vi "Autonomous Independent.vi"   [LabVIEW 2019]
doc: "This VI is called when autonomous begins, and will automatically be terminated when autonomous ends. You can carry out timed or sensor driven robot movement independently without needing to return to the caller."
uses:
  <vilib>/Utility/file.llb/Read Delimited Spreadsheet (string).vi
  RobotGlobal.vi
  Classes/Robot/Panzer/Panzer.lvclass
panel:
  # "Be sure to right-click and choose Data Operations>>Make Current Value default if you want to save the array values with the VI"
types:
  T1 = typedef "RobotObjects.ctl" = cluster{"Drive.lvclass":refnum<class "Tank Drive.lvclass">, "Pneumatics.lvclass":refnum<class "Pneumatics.lvclass">, "Vision.lvclass":refnum<class "Vision.lvclass">, "Joysticks.lvclass":refnum<class "Joysticks.lvclass">, "Elevator.lvclass":refnum<class "Elevator.lvclass">, "Hatch.lvclass":refnum<class "Hatch.lvclass">, "Cargo.lvclass":refnum<class "Cargo.lvclass">, "DriveOld.lvclass":refnum<class "Drive.lvclass">, "Robot.lvclass":refnum<class "Robot.lvclass">, "Control Panel.lvclass":refnum<class "Control Panel.lvclass">, "Climber.lvclass":refnum<class "Climber.lvclass">, "Turret.lvlib:Turret.lvclass":refnum<class "Turret.lvclass">, "Power Cell Handler.lvclass":refnum<class "Power Cell Handler.lvclass">}
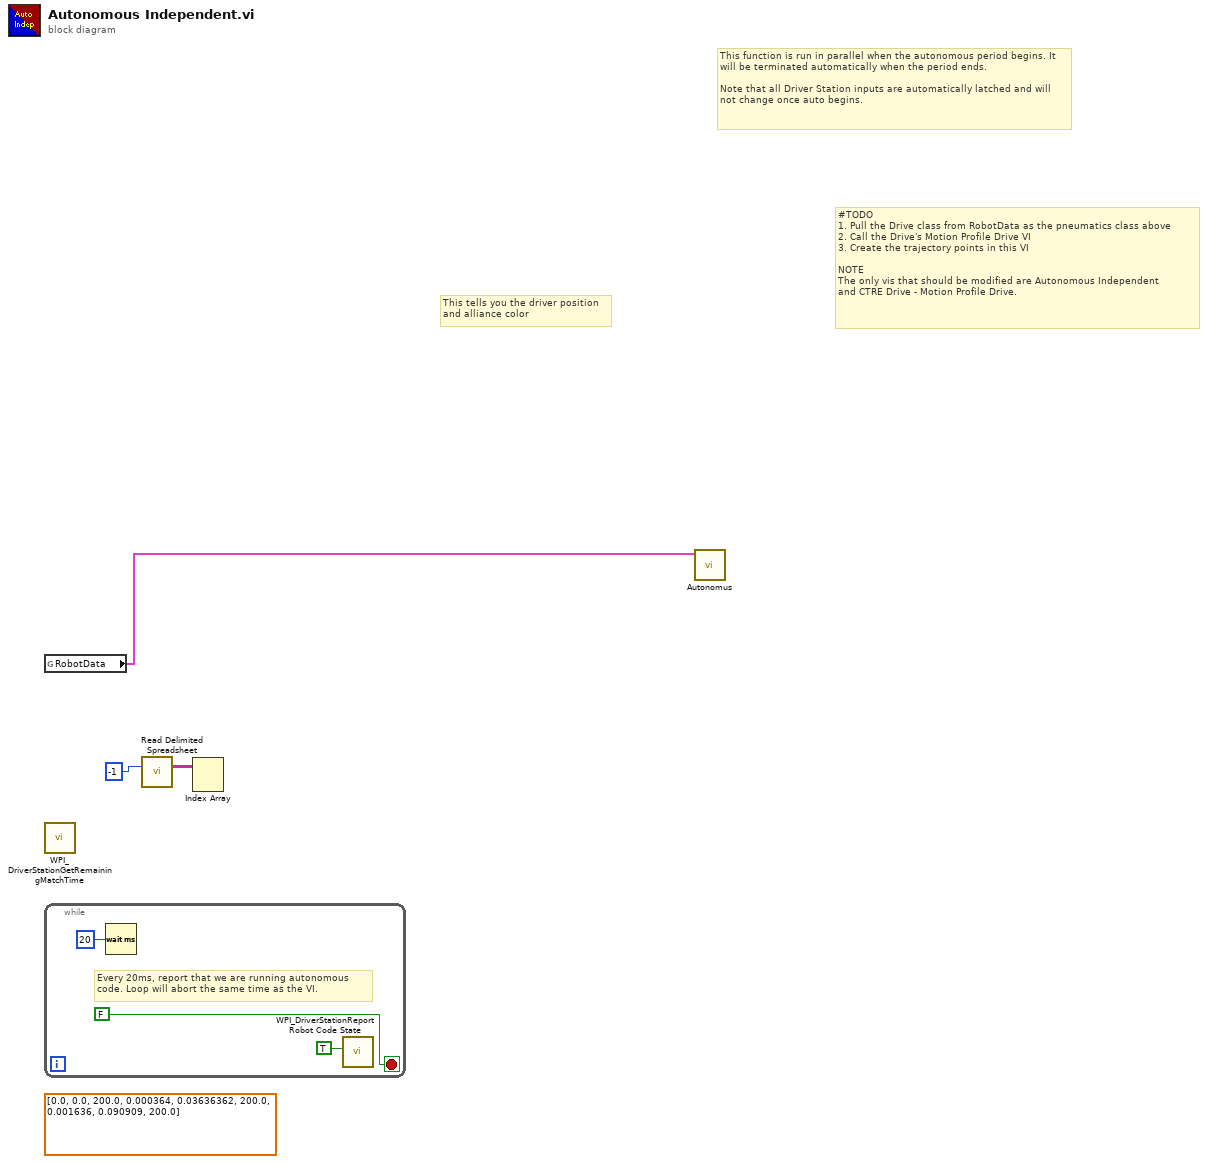
[diagram p0: block diagram]
diagram:
  (unwired) dbl[][] [[0.0, 0.0, 200.0], [0.000364, 0.03636362, 200.0], [0.001636, 0.090909, 200.0]] ("all rows")
  # "#TODO\n1. Pull the Drive class from RobotData as the pneumatics class above\n2. Call the Drive's Motion Profile Drive VI\n3. Create the trajectory points in this VI\n\nNOTE\nThe only vis that should be modified are Autonomous Independent \nand CTRE Drive - Motion Profile Drive."
  # "This function is run in parallel when the autonomous period begins. It will be terminated automatically when the period ends.\n\nNote that all Driver Station inputs are automatically latched and will not change once auto begins."
  # "This tells you the driver position\nand alliance color"
  n1 = global read "RobotGlobal.vi" "RobotData"() -> (w1:T1)
  n2 = call <vilib>:"WPI_DriverStationGetRemainingMatchTime.vi"() -> ()  [unwired: 10 in, 2 out]
  n3 = while {
    stop <- FALSE stop-if-true
    # "Every 20ms, report that we are running autonomous\ncode. Loop will abort the same time as the VI."
    n4 = Wait (ms)(milliseconds to wait=u32 20) -> ()  [unwired: 1 out]
    n5 = call <vilib>:"WPI_DriverStationReport Robot Code State.vi"("Autonomous"=TRUE) -> ()  [unwired: 10 in, 1 out]
  }
  n6 = call-poly <vilib>:"Read Delimited Spreadsheet.vi"("number of rows (all:-1)"=-1) -> ("all rows"=w2:string[][])  [unwired: 9 in, 5 out]
  n7 = Index Array(array=w2) -> ()  [unwired: 2 in, 1 out]
  n8 = call "Autonomus.vi"("RobotData"=w1) -> ()  [unwired: 11 in]
